vi "InitVars.vi"(8 "error in (no error)":errorcluster caption="Fehler (Eingang, kein Fehler)") -> (0 "error out":errorcluster caption="Fehler (Ausgang)")   [LabVIEW 2014]
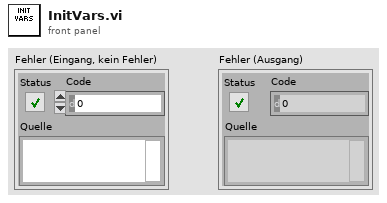
[diagram p1: front panel]
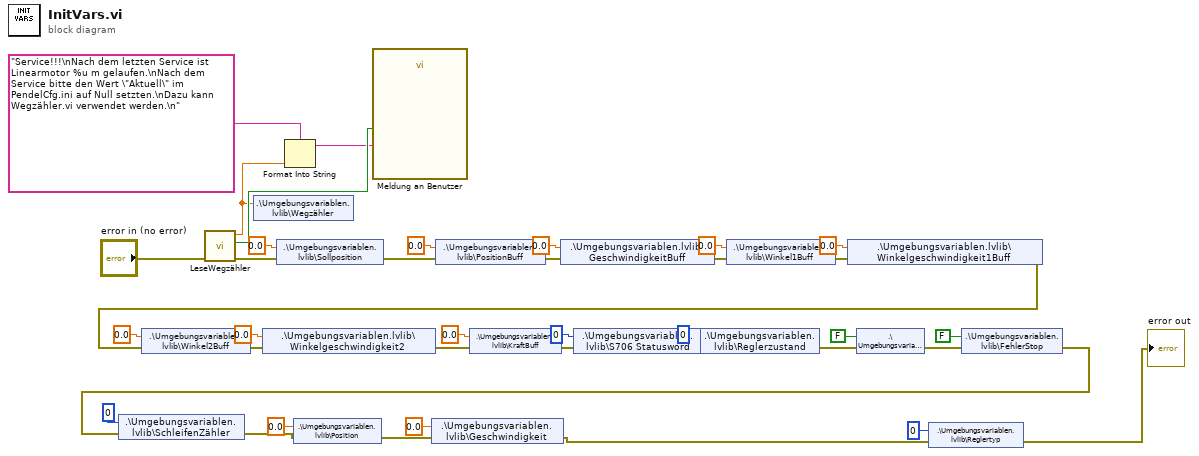
[diagram p0: block diagram]
diagram:
  n1 = call "LeseWegzähler.vi"("error in (no error)"="error in (no error)") -> ("error out"=w13:errorcluster, "Zeit für Service"=w22:bool, "value"=w21:dbl)  [unwired: 8 in]
  n2 = shared-variable ".\\Umgebungsvariablen.lvlib\\Wegzähler"(w21) -> ()  [unwired: 1 in, 1 out]
  n3 = shared-variable ".\\Umgebungsvariablen.lvlib\\Sollposition"(0.0 ("Sollposition"), error in=w13) -> (error out=w12:errorcluster)
  n4 = Format Into String(format string="Service!!!\nNach dem letzten Service ist Linearmotor %u m gelaufen.\nNach dem Service bitte den Wert \"Aktuell\" im PendelCfg.ini auf Null setzten.\nDazu kann Wegzähler.vi verwendet werden.\n" ("Eingangs-String"), w21) -> (resulting string=w19:string)  [unwired: 2 in, 1 out]
  n5 = call "Meldung an Benutzer"("Enable"=w22, "Message"=w19) -> ()  [unwired: 8 in, 2 out]
  n6 = shared-variable ".\\Umgebungsvariablen.lvlib\\PositionBuff"(0.0 ("Position"), error in=w12) -> (error out=w38:errorcluster)
  n7 = shared-variable ".\\Umgebungsvariablen.lvlib\\GeschwindigkeitBuff"(0.0 ("Geschwindigkeit"), error in=w38) -> (error out=w37:errorcluster)
  n8 = shared-variable ".\\Umgebungsvariablen.lvlib\\Winkel1Buff"(0.0 ("Winkel1"), error in=w37) -> (error out=w36:errorcluster)
  n9 = shared-variable ".\\Umgebungsvariablen.lvlib\\Winkelgeschwindigkeit1Buff"(0.0 ("Winkel1"), error in=w36) -> (error out=w26:errorcluster)
  n10 = shared-variable ".\\Umgebungsvariablen.lvlib\\Winkel2Buff"(0.0 ("Winkelgeschwindigkeit1"), error in=w26) -> (error out=w27:errorcluster)
  n11 = shared-variable ".\\Umgebungsvariablen.lvlib\\Winkelgeschwindigkeit2"(0.0 ("Winkel2"), error in=w27) -> (error out=w11:errorcluster)
  n12 = shared-variable ".\\Umgebungsvariablen.lvlib\\KraftBuff"(0.0 ("Kraft"), error in=w11) -> (error out=w10:errorcluster)
  n13 = shared-variable ".\\Umgebungsvariablen.lvlib\\S706 Statusword"(u16 0 ("SR Status"), error in=w10) -> (error out=w17:errorcluster)
  n14 = shared-variable ".\\Umgebungsvariablen.lvlib\\Reglerzustand"(u16 0 ("Reglerzustand"), error in=w17) -> (error out=w28:errorcluster)
  n15 = shared-variable ".\\Umgebungsvariablen.lvlib\\stop"(FALSE ("stop"), error in=w28) -> (error out=w23:errorcluster)
  n16 = shared-variable ".\\Umgebungsvariablen.lvlib\\FehlerStop"(FALSE ("FehlerStop"), error in=w23) -> (error out=w6:errorcluster)
  n17 = shared-variable ".\\Umgebungsvariablen.lvlib\\SchleifenZähler"(u16 0 ("SchleifenZähler"), error in=w6) -> (error out=w5:errorcluster)
  n18 = shared-variable ".\\Umgebungsvariablen.lvlib\\Position"(0.0 ("Position"), error in=w5) -> (error out=w4:errorcluster)
  n19 = shared-variable ".\\Umgebungsvariablen.lvlib\\Geschwindigkeit"(0.0 ("Geschwindigkeit"), error in=w4) -> (error out=w1:errorcluster)
  n20 = shared-variable ".\\Umgebungsvariablen.lvlib\\Reglertyp"(i16 0 ("Reglertyp"), error in=w1) -> (error out=→"error out":errorcluster)
